vi "Update.vi"(8 "error in (no error)":errorcluster, 11 "Joystick in":refnum<class "Joystick.lvclass">) -> (0 "error out":errorcluster, 3 "Joystick out":refnum<class "Joystick.lvclass">)   [LabVIEW 2020, in "Joystick.lvlib" / "Joystick.lvclass"]
uses:
  Joystick.lvclass
  Joystick.lvclass/Joystick.ctl
  <vilib>/Utility/inputDevices.llb/joystickAcquire.vi
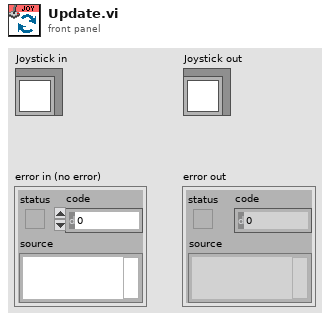
[diagram p1: front panel]
types:
  T1 = cluster{"X axis":i32, "Y axis":i32, "Z axis":i32, "X axis rotation":i32, "Y axis rotation":i32, "Z axis rotation":i32, "U axis":i32, "V axis":i32}
  T2 = cluster{"button 1":bool, "button 2":bool, "button 3":bool, "button 4":bool, "button 5":bool, "button 6":bool, "button 7":bool, "button 8":bool, "button 9":bool, "button 10":bool, "button 11":bool, "button 12":bool, "button 13":bool, "button 14":bool, "button 15":bool, "button 16":bool, "button 17":bool, "button 18":bool, "button 19":bool, "button 20":bool, "button 21":bool, "button 22":bool, "button 23":bool, "button 24":bool, "button 25":bool, "button 26":bool, "button 27":bool, "button 28":bool, "button 29":bool, "button 30":bool, "button 31":bool, "button 32":bool}
  T3 = cluster{"pov 1":i32, "pov 2":i32, "pov 3":i32, "pov 4":i32}
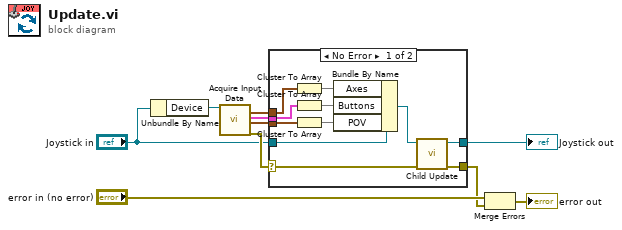
[diagram p0: block diagram]
diagram:
  n1 = Unbundle By Name("Joystick in") -> ("Device"=w10:refnum<k1>)
  n2 = call-poly <vilib>:"Acquire Input Data.vi"("device ID"=w10) -> ("axis info"=w6:T1, "button info"=w7:T2, "direction info"=w8:T3, "error out"=w9:errorcluster)  [unwired: 14 in, 1 out]
  n3 = case shown="No Error" w9 {
    selector: w9 -> [w11 w22]
    tunnel: w8 -> [w19 _]
    tunnel: w7 -> [w20 _]
    tunnel: w6 -> [w21 _]
    tunnel: "Joystick in" -> [w18 w23]
    tunnel: [w14 w23] -> w4
    tunnel: [w12 w22] -> w2
    frame No Error {
      n4 = Cluster To Array(cluster=w21) -> (array=w15:i32[])
      n5 = Cluster To Array(cluster=w20) -> (array=w16:bool[])
      n6 = Cluster To Array(cluster=w19) -> (array=w17:i32[])
      n7 = Bundle By Name(cluster=w18, "Axes"=w15, "Buttons"=w16, "POV"=w17) -> (w13:refnum<class "Joystick.lvclass">)
      n8 = call-dynamic "Child Update.vi"("error in (no error)"=w11, "Joystick in"=w13) -> ("error out"=w12:errorcluster, "Joystick out"=w14:refnum<class "Joystick.lvclass">)  [unwired: 8 in]
    }
    frame Error {
    }
  }
  "Joystick out" <- w4
  n9 = Merge Errors("error in (no error)", w2) -> (→"error out":errorcluster)
